vi "Initialize Actor.vi"(7 "Host Name":string, 8 "error in (no error)":errorcluster, 9 "Actor Name":string, 10 "Message Broker Interface":refnum<class "Message Broker Interface.lvclass">, 11 "Terminal Message in":refnum<class "Terminal Message.lvclass">) -> (0 "error out":errorcluster, 3 "Terminal Message out":refnum<class "Terminal Message.lvclass">)   [LabVIEW 2016, in "CLD Exam - ATM.lvlib" / "Terminal Message.lvclass"]
uses:
  Terminal Message.lvclass
  Mediator/Classes/Message Broker Interface/Message Broker Interface.lvclass
  Terminal Message.lvclass/Terminal Message.ctl
  Mediator/Classes/Message Transport Event/Message Transport Event.lvclass
  D:/Repos/Stream/software/Mediator/Classes/Message Transport Interface/Message Transport Interface.lvclass
  Mediator/Classes/Mediated Synchronous Actor/Mediated Synchronous Actor.lvclass
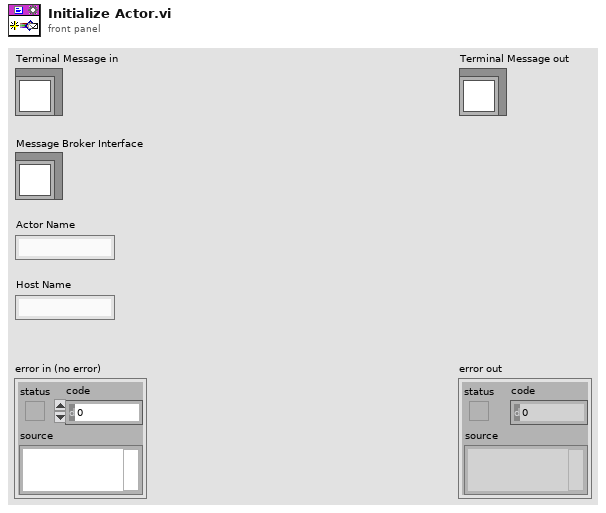
[diagram p1: front panel]
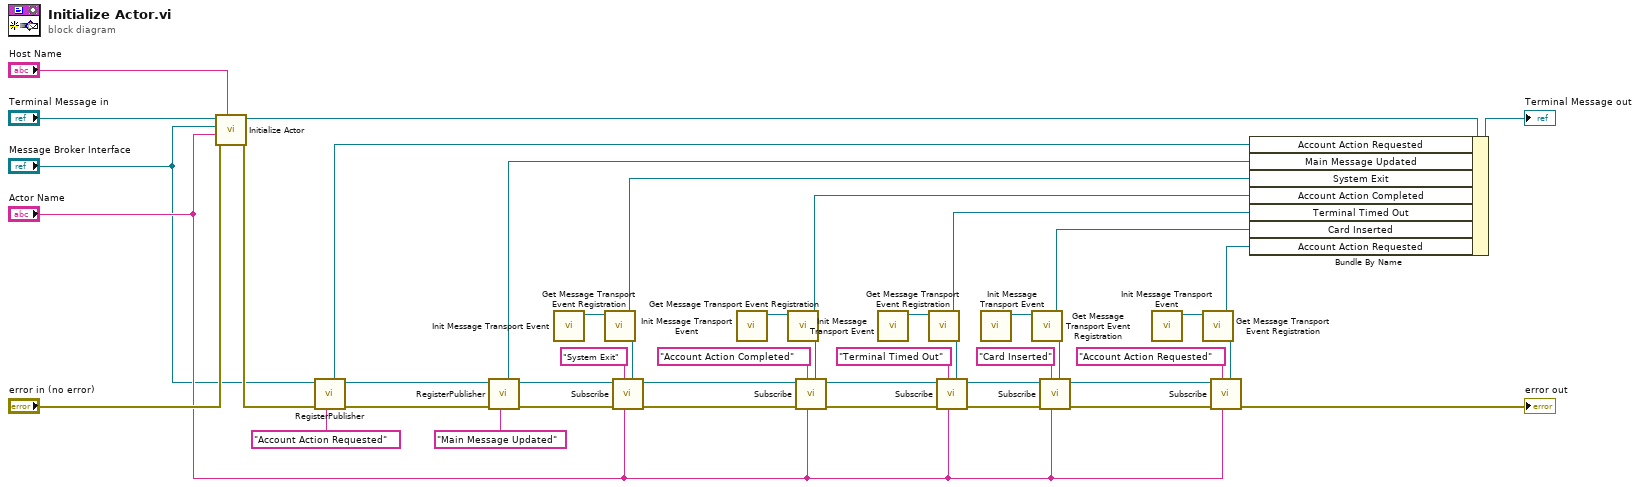
[diagram p0: block diagram]
diagram:
  n1 = call-parent "Initialize Actor.vi"("Host Name"="Host Name", "error in (no error)"="error in (no error)", "Actor Name"="Actor Name", "Message Broker Interface"="Message Broker Interface", "Mediated Synchronous Actor in"="Terminal Message in") -> ("error out"=w11:errorcluster, "Mediated Synchronous Actor out"=w42:refnum<class "Terminal Message.lvclass">)  [unwired: 5 in]
  n2 = call-dynamic "RegisterPublisher.vi"("Topic Name"="Account Action Requested", "error in (no error)"=w11, "Message Broker Interface in"="Message Broker Interface") -> ("error out"=w10:errorcluster, "Message Broker Interface out"=w8:refnum<class "Message Broker Interface.lvclass">, "Transport"=w7:refnum<class "Message Transport Queue.lvclass">)  [unwired: 4 in, 2 out]
  n3 = call-dynamic "RegisterPublisher.vi"("Topic Name"="Main Message Updated", "error in (no error)"=w10, "Message Broker Interface in"=w8) -> ("error out"=w5:errorcluster, "Message Broker Interface out"=w6:refnum<class "Message Broker Interface.lvclass">, "Transport"=w35:refnum<class "Message Transport Queue.lvclass">)  [unwired: 4 in, 2 out]
  n4 = call "Init Message Transport Event.vi"() -> ("Message Transport Event out"=w40:refnum<class "Message Transport Event.lvclass">)  [unwired: 10 in, 1 out]
  n5 = call "Get Message Transport Event Registration.vi"("Message Transport Event in"=w40) -> ("Event Registration Refnum"=w37:refnum<event-registration>, "Message Transport Event out"=w39:refnum<class "Message Transport Event.lvclass">)  [unwired: 7 in, 2 out]
  n6 = call-dynamic "Subscribe.vi"("Message Transport Interface"=w39, "Subscriber Name"="Actor Name", "Topic Name"="System Exit", "error in (no error)"=w5, "Message Broker Interface in"=w6) -> ("error out"=w3:errorcluster, "Message Broker Interface out"=w4:refnum<class "Message Broker Interface.lvclass">)  [unwired: 4 in, 1 out]
  n7 = call "Init Message Transport Event.vi"() -> ("Message Transport Event out"=w34:refnum<class "Message Transport Event.lvclass">)  [unwired: 10 in, 1 out]
  n8 = call "Get Message Transport Event Registration.vi"("Message Transport Event in"=w34) -> ("Event Registration Refnum"=w31:refnum<event-registration>, "Message Transport Event out"=w33:refnum<class "Message Transport Event.lvclass">)  [unwired: 7 in, 2 out]
  n9 = call-dynamic "Subscribe.vi"("Message Transport Interface"=w33, "Subscriber Name"="Actor Name", "Topic Name"="Account Action Completed", "error in (no error)"=w3, "Message Broker Interface in"=w4) -> ("error out"=w1:errorcluster, "Message Broker Interface out"=w2:refnum<class "Message Broker Interface.lvclass">)  [unwired: 4 in, 1 out]
  n10 = call "Init Message Transport Event.vi"() -> ("Message Transport Event out"=w30:refnum<class "Message Transport Event.lvclass">)  [unwired: 10 in, 1 out]
  n11 = call "Get Message Transport Event Registration.vi"("Message Transport Event in"=w30) -> ("Event Registration Refnum"=w27:refnum<event-registration>, "Message Transport Event out"=w29:refnum<class "Message Transport Event.lvclass">)  [unwired: 7 in, 2 out]
  n12 = call-dynamic "Subscribe.vi"("Message Transport Interface"=w29, "Subscriber Name"="Actor Name", "Topic Name"="Terminal Timed Out", "error in (no error)"=w1, "Message Broker Interface in"=w2) -> ("error out"=w23:errorcluster, "Message Broker Interface out"=w22:refnum<class "Message Broker Interface.lvclass">)  [unwired: 4 in, 1 out]
  n13 = call "Init Message Transport Event.vi"() -> ("Message Transport Event out"=w24:refnum<class "Message Transport Event.lvclass">)  [unwired: 10 in, 1 out]
  n14 = call "Get Message Transport Event Registration.vi"("Message Transport Event in"=w24) -> ("Event Registration Refnum"=w21:refnum<event-registration>, "Message Transport Event out"=w25:refnum<class "Message Transport Event.lvclass">)  [unwired: 7 in, 2 out]
  n15 = call-dynamic "Subscribe.vi"("Message Transport Interface"=w25, "Subscriber Name"="Actor Name", "Topic Name"="Card Inserted", "error in (no error)"=w23, "Message Broker Interface in"=w22) -> ("error out"=w15:errorcluster, "Message Broker Interface out"=w17:refnum<class "Message Broker Interface.lvclass">)  [unwired: 4 in, 1 out]
  n16 = call "Init Message Transport Event.vi"() -> ("Message Transport Event out"=w20:refnum<class "Message Transport Event.lvclass">)  [unwired: 10 in, 1 out]
  n17 = call "Get Message Transport Event Registration.vi"("Message Transport Event in"=w20) -> ("Event Registration Refnum"=w14:refnum<event-registration>, "Message Transport Event out"=w19:refnum<class "Message Transport Event.lvclass">)  [unwired: 7 in, 2 out]
  n18 = call-dynamic "Subscribe.vi"("Message Transport Interface"=w19, "Subscriber Name"="Actor Name", "Topic Name"="Account Action Requested", "error in (no error)"=w15, "Message Broker Interface in"=w17) -> ("error out"=→"error out":errorcluster)  [unwired: 4 in, 2 out]
  n19 = Bundle By Name(cluster=w42, "Account Action Requested"=w7, "Main Message Updated"=w35, "System Exit"=w37, "Account Action Completed"=w31, "Terminal Timed Out"=w27, "Card Inserted"=w21, "Account Action Requested"=w14) -> (→"Terminal Message out":refnum<class "Terminal Message.lvclass">)
